vi "get Player Type.vi"(11 "Element in":refnum<class "Element.lvclass">) -> (3 "Player Type":T1)   [LabVIEW 2021, in "Element.lvclass"]
uses:
  Element.lvclass
  Element.lvclass/Element.ctl
  Player Type.ctl
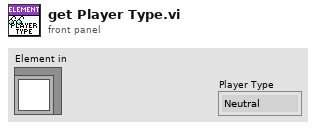
[diagram p1: front panel]
types:
  T1 = typedef "Element.lvclass/Player Type.ctl" = enum16{"Neutral", "Player 1", "Player 2"}
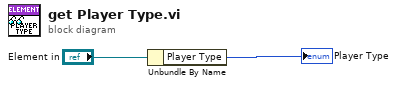
[diagram p0: block diagram]
diagram:
  n1 = Unbundle By Name("Element in") -> ("Player Type"=→"Player Type":T1)
